vi "ZeroMQ Device Shot Client.vi"(10 "device port":u16, 11 "MCaddress":u32) -> ()   [LabVIEW 2020]
uses:
  <vilib>/addons/zeromq/socket_type.ctl
  <vilib>/addons/zeromq/socket_options.ctl
  shared/stop FGV control.ctl
  UDPComm/UDP FGV control.ctl
  shared/BasicFGV_control.ctl
  shared/UDP_FGV.ctl
  <vilib>/addons/zeromq/zmq_context.lvclass
  <vilib>/addons/zeromq/zeromq.lvlib
  <vilib>/addons/zeromq/zmq_socket.lvclass
  UDPComm/UDPComm.lvlib
panel:
  in  "ZeroMQ (MC) port":i32=5555
  out "error out":errorcluster
  out "timeout?":bool
  out "messages":string[](array[string])
  out "# scan ends 2":i32
  out "last scan end 2":string
  out "last unrec cmd 2":string
  out "Last shot path 2":string
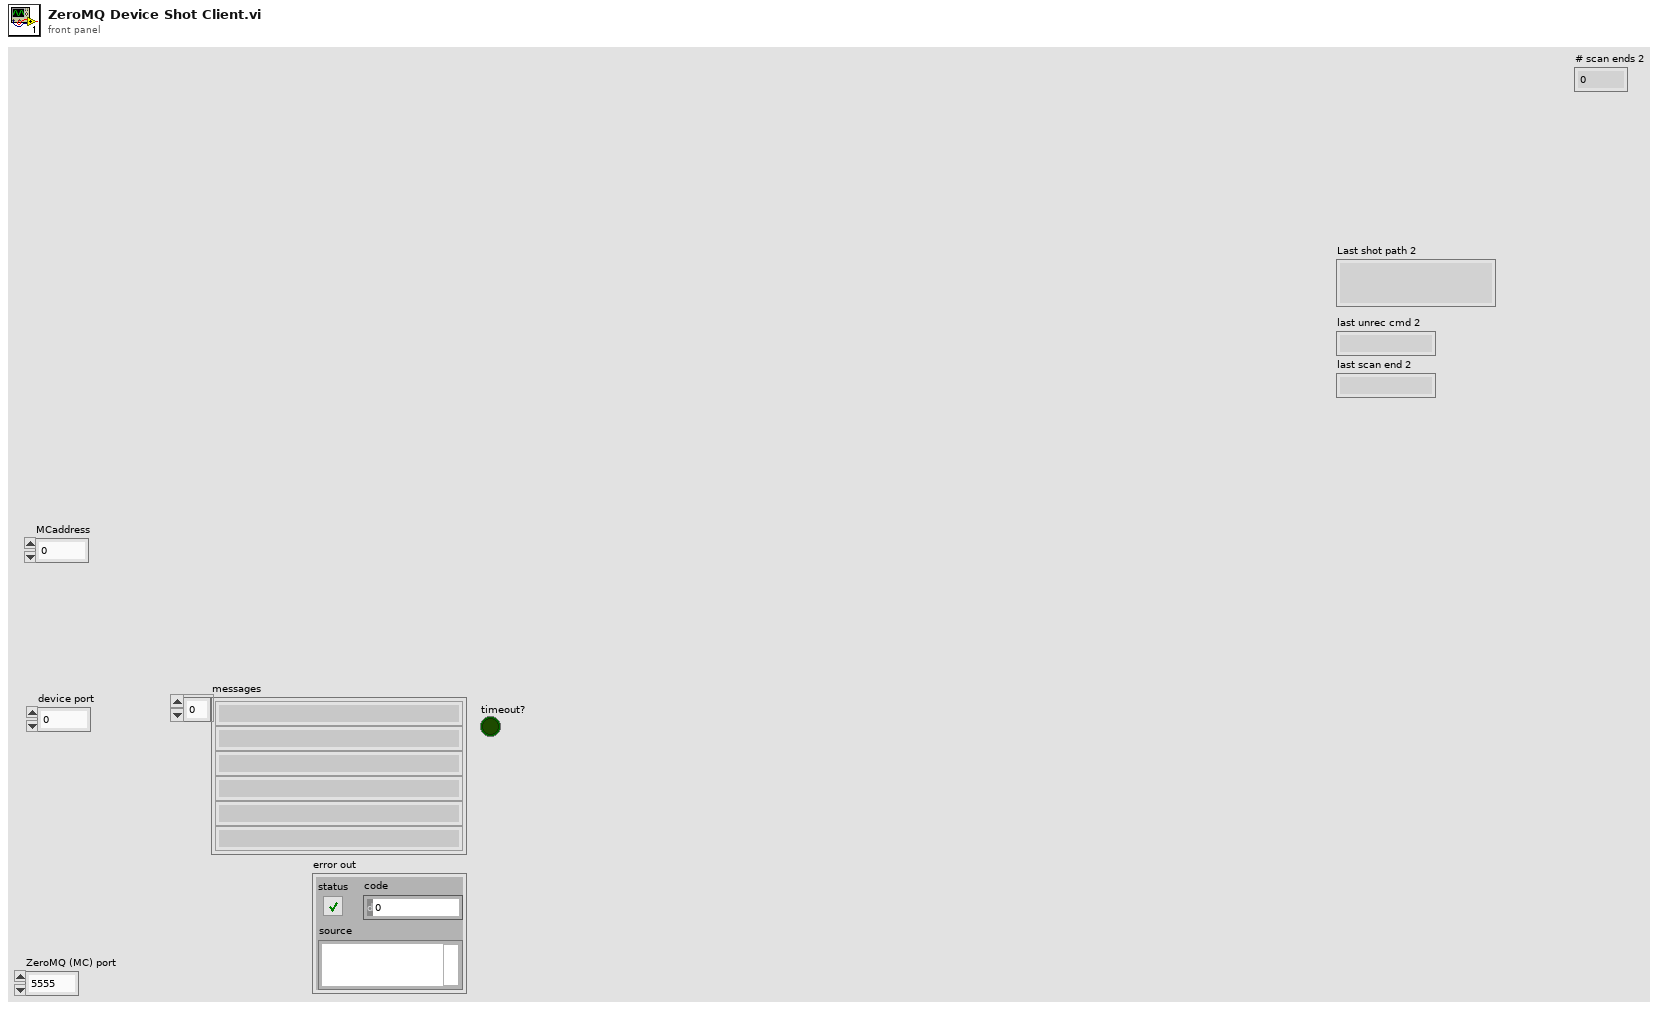
[diagram p1: front panel]
types:
  T1 = typedef "zeromq.lvlib/socket_options.ctl" = enum8{"NONE", "ZMQ_HWM", "<2>", "ZMQ_SWAP", "ZMQ_AFFINITY", "ZMQ_ROUTING_ID", "ZMQ_SUBSCRIBE", "ZMQ_UNSUBSCRIBE", "ZMQ_RATE", "ZMQ_RECOVERY_IVL", "ZMQ_MCAST_LOOP", "ZMQ_SNDBUF", "ZMQ_RCVBUF", "ZMQ_RCVMORE", "ZMQ_FD", "ZMQ_EVENTS", "ZMQ_TYPE", "ZMQ_LINGER", "ZMQ_RECONNECT_IVL", "ZMQ_BACKLOG", "ZMQ_RECOVERY_IVL_MSEC", "ZMQ_RECONNECT_IVL_MAX", "ZMQ_MAXMSGSIZE", "ZMQ_SNDHWM", "ZMQ_RCVHWM", "ZMQ_MULTICAST_HOPS", "<26>", "ZMQ_RCVTIMEO", "ZMQ_SNDTIMEO", "<29>", "<30>", "ZMQ_IPV4ONLY", "ZMQ_LAST_ENDPOINT", "ZMQ_ROUTER_MANDATORY", "ZMQ_TCP_KEEPALIVE", "ZMQ_TCP_KEEPALIVE_CNT", "ZMQ_TCP_KEEPALIVE_IDLE", "ZMQ_TCP_KEEPALIVE_INTVL", "ZMQ_TCP_ACCEPT_FILTER", "ZMQ_IMMEDIATE", "ZMQ_XPUB_VERBOSE", "ZMQ_ROUTER_RAW", "ZMQ_IPV6", "ZMQ_MECHANISM", "ZMQ_PLAIN_SERVER", "ZMQ_PLAIN_USERNAME", "ZMQ_PLAIN_PASSWORD", "ZMQ_CURVE_SERVER", "ZMQ_CURVE_PUBLICKEY", "ZMQ_CURVE_SECRETKEY", "ZMQ_CURVE_SERVERKEY", "ZMQ_PROBE_ROUTER", "ZMQ_REQ_CORRELATE", "ZMQ_REQ_RELAXED", "ZMQ_CONFLATE", "ZMQ_ZAP_DOMAIN", "ZMQ_ROUTER_HANDOVER", "ZMQ_TOS", "ZMQ_IPC_FILTER_PID", "ZMQ_IPC_FILTER_UID", "ZMQ_IPC_FILTER_GID", "ZMQ_CONNECT_ROUTING_ID", "ZMQ_GSSAPI_SERVER", "ZMQ_GSSAPI_PRINCIPAL", "ZMQ_GSSAPI_SERVICE_PRINCIPAL", "ZMQ_GSSAPI_PLAINTEXT", "ZMQ_HANDSHAKE_IVL", "<67>", "ZMQ_SOCKS_PROXY", "ZMQ_XPUB_NODROP", "ZMQ_BLOCKY", "ZMQ_XPUB_MANUAL", "ZMQ_XPUB_WELCOME_MSG", "ZMQ_STREAM_NOTIFY", "ZMQ_INVERT_MATCHING", "ZMQ_HEARTBEAT_IVL", "ZMQ_HEARTBEAT_TTL", "ZMQ_HEARTBEAT_TIMEOUT", "ZMQ_XPUB_VERBOSER", "ZMQ_CONNECT_TIMEOUT", "ZMQ_TCP_MAXRT", "ZMQ_THREAD_SAFE", "<82>", "<83>", "ZMQ_MULTICAST_MAXTPDU", "ZMQ_VMCI_BUFFER_SIZE", "ZMQ_VMCI_BUFFER_MIN_SIZE", "ZMQ_VMCI_BUFFER_MAX_SIZE", "ZMQ_VMCI_CONNECT_TIMEOUT", "ZMQ_USE_FD", "ZMQ_GSSAPI_PRINCIPAL_NAMETYPE", "ZMQ_GSSAPI_SERVICE_PRINCIPAL_NAMETYPE", "ZMQ_BINDTODEVICE", "ZMQ_ZAP_ENFORCE_DOMAIN", "ZMQ_LOOPBACK_FASTPATH", "ZMQ_METADATA", "ZMQ_MULTICAST_LOOP", "ZMQ_ROUTER_NOTIFY"}
  T2 = typedef "zeromq.lvlib/socket_type.ctl" = enum8{"ZMQ_PAIR", "ZMQ_PUB", "ZMQ_SUB", "ZMQ_REQ", "ZMQ_REP", "ZMQ_DEALER", "ZMQ_ROUTER", "ZMQ_PULL", "ZMQ_PUSH", "ZMQ_XPUB", "ZMQ_XSUB", "ZMQ_STREAM", "ZMQ_SERVER", "ZMQ_CLIENT", "ZMQ_RADIO", "ZMQ_DISH", "ZMQ_GATHER", "ZMQ_SCATTER", "ZMQ_DGRAM"}
  T3 = typedef "stop FGV control.ctl" = enum16{"Clear", "Write", "Read"}
  T4 = typedef "UDP_FGV.ctl" = cluster{"address":u32, "port":u16, "data":string, "Busy":bool, "response":string, "imm response":string, "MC IP":string}
  T5 = typedef "BasicFGV_control.ctl" = enum16{"get", "set", "reset"}
  T6 = typedef "UDP FGV control.ctl" = enum16{"Clear", "WriteToSM", "ReadFromSM", "WriteToUDP", "ReadFromUDP", "LockIP", "UnLockIP"}
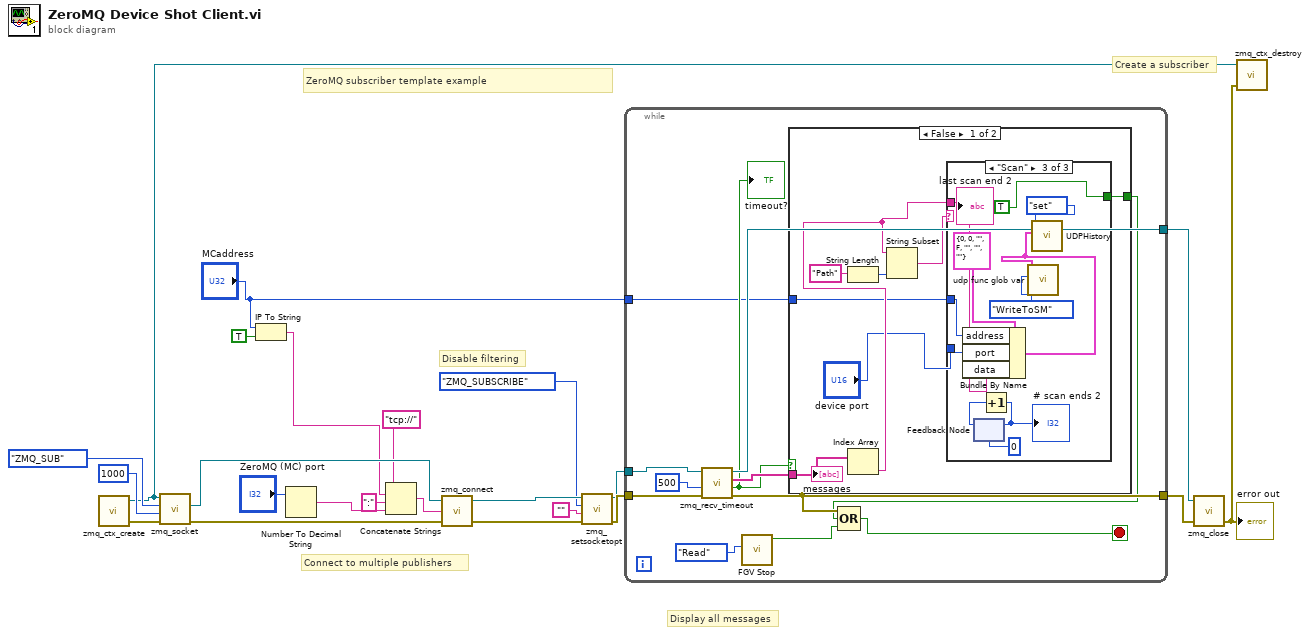
[diagram p0: block diagram]
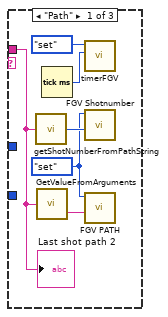
[diagram p2: hidden frame]
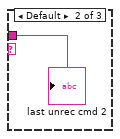
[diagram p3: hidden frame]
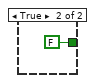
[diagram p4: hidden frame]
diagram:
  # "ZeroMQ subscriber template example"
  # "Display all messages"
  # "Create a subscriber"
  # "Disable filtering"
  # "Connect to multiple publishers"
  n1 = call <vilib>:"zmq_ctx_create.vi"() -> ("error out"=w22:errorcluster, "context out"=w13:refnum<class "zmq_context.lvclass">)  [unwired: 4 in]
  n2 = call <vilib>:"zmq_socket.vi"("error in"=w22, "linger (ms)"=1000, "socket type"=socket_type."ZMQ_SUB", "context in"=w13) -> ("error out"=w21:errorcluster, "socket out"=w15:refnum<class "zmq_socket.lvclass">)  [unwired: 1 in, 1 out]
  n3 = IP To String(1:TRUE ("dot notation? (F)"), 2:"MCaddress") -> (0:w3:string)
  n4 = Number To Decimal String(number="ZeroMQ (MC) port") -> (decimal integer string=w7:string)  [unwired: 1 in]
  n5 = Concatenate Strings("tcp://" ("string"), w3, ":" ("string"), w7) -> (w8:string)
  n6 = call <vilib>:"zmq_connect.vi"("error in"=w21, "endpoint"=w8, "socket in"=w15) -> ("error out"=w19:errorcluster, "socket out"=w20:refnum<class "zmq_socket.lvclass">)  [unwired: 1 in]
  n7 = call <vilib>:"zmq_setsocketopt.vi"("error in"=w19, "value"="", "option"=socket_options."ZMQ_SUBSCRIBE", "socket in"=w20) -> ("error out"=w18:errorcluster, "socket out"=w12:refnum<class "zmq_socket.lvclass">)  [unwired: 2 in]
  n8 = while {
    tunnel: w12 -> [w35]
    tunnel: w18 -> [w34]
    tunnel: [w29] -> w10
    tunnel: [w32] -> w11
    tunnel: "MCaddress" -> [w24]
    stop <- w28 stop-if-true
    n9 = call <vilib>:"zmq_recv_timeout.vi"("error in"=w34, "timeout (ms)"=u32 500, "socket in"=w35) -> ("error out"=w29:errorcluster, "timeout?"=w30:bool, "parts"=w31:string[], "socket out"=w32:refnum<class "zmq_socket.lvclass">)  [unwired: 1 in]
    "timeout?" <- w30
    n10 = call "FGV Stop.vi"("Function"=stop_FGV_control."Read") -> ("stop out"=w25:bool)  [unwired: 9 in, 1 out]
    n11 = case shown="False" w30 {
      tunnel: w31 -> [w43 _]
      tunnel: [w38 FALSE] -> w26
      tunnel: w24 -> [w37 _]
      frame False {
        n12 = String Length(string="Path" ("Command")) -> (length=w41:i32)
        n13 = Index Array(array=w43) -> (element=w39:string)  [unwired: 1 in]
        n14 = String Subset(string=w39, length (rest)=w41) -> (substring=w42:string)  [unwired: 1 in]
        n15 = case shown="\"Scan\"" w42 {
          tunnel: w39 -> [w44 w50 w57]
          tunnel: [_ _ TRUE] -> w38
          tunnel: w37 -> [_ _ w59]
          tunnel: "device port" -> [_ _ w58]
          frame "Path" {
            w45 = enum16{"set", "get", "reset"}."set" ("command")
            n16 = call "getShotNumberFromPathString.vi"("Path String"=w44) -> ("ShotNumber from path"=w47:i32)
            n17 = call "GetValueFromArguments.vi"("Arguments"=w44) -> ("Ip:port"=w48:string)  [unwired: 1 out]
            n18 = Tick Count (ms)() -> (millisecond timer value=w49:u32)
            n19 = call "timerFGV.vi"("millisecond timer value"=w49, "command"=enum16{"set", "get", "reset"}."set") -> ()  [unwired: 9 in, 1 out]
            n20 = call "FGV Shotnumber.vi"("shot#"=w47, "command"=w45) -> ()  [unwired: 7 in, 3 out]
            n21 = call "FGV PATH.vi"("Saving Path (UDP)"=w48, "command"=w45) -> ()  [unwired: 9 in, 1 out]
            "Last shot path 2" <- w44
          }
          frame Default {
            "last unrec cmd 2" <- w50
          }
          frame "Scan" {
            n22 = Bundle By Name(cluster=T4 {"address"=0, "port"=0, "data"="", "Busy"=FALSE, "response"="", "imm response"="", "MC IP"=""} ("UDPFGV"), "address"=w59, "port"=w58, "data"=w57) -> (w56:T4)
            n23 = feedback #1(0) -> (w52:i32)
            n24 = Increment(x=w52) -> (x+1=w53:i32)
            "# scan ends 2" <- w53
            n25 = feedback-in #1(w53) -> ()
            n26 = call "udp func glob var.vi"("Function"=UDP_FGV_control."WriteToSM", "Msg in"=w56) -> ()  [unwired: 7 in, 3 out]
            n27 = call "UDPHistory.vi"("UDPFGV"=w56, "command"=BasicFGV_control."set") -> ()  [unwired: 9 in, 1 out]
            "last scan end 2" <- w57
          }
        }
        "messages" <- w43
      }
      frame True {
      }
    }
    n28 = Compound Arithmetic op=OR(w29, w26, w25) -> (w28:bool)
  }
  n29 = call <vilib>:"zmq_close.vi"("error in"=w10, "socket"=w11) -> ("error out"=w9:errorcluster)  [unwired: 3 in]
  "error out" <- w9
  n30 = call <vilib>:"zmq_ctx_destroy.vi"("error in"=w9, "context in"=w13) -> ()  [unwired: 3 in, 1 out]
